vi "Live Capture Functional Stack.vi"() -> ()   [LabVIEW 2013]
uses:
  subvis/Stack Track.ctl
  subvis/Stack_State.ctl
panel:
  in  "Internal Line Interval":dbl
  in  "Slit Width / Lines":sgl=150.0
  in  "Camera Readout Mode":u16(ring)=12 items=["Full Frame"=1, "Slit Scanning"=12]
  in  "Readout Direction":sgl(ring)=1.0 items=["Forward"=1, "Backward"=2]
  in  "Trigger Mode":sgl(ring)=1.0 items=["Normal"=1, "Start "=6]
  in  "Trigger Source":sgl(ring)=2.0 items=["Internal"=1, "External"=2]
  out "Enum":T1
  out "Image":u16[][](graph)
  out "Saving":bool
  in  "AutoIncrement":bool=TRUE
  in  "Path":path=path "C:/Users/spim/Desktop/Craig Cap/temp/a.tiff"
  in  "Frames":i32=100
  out "Frame Index":i32
  out "error out":errorcluster
  in  "stop":bool
  in  "Capture":bool
  out "Total Frames":i32
  out "Elapsed Time":u32
  out "Software FPS":dbl
  out "Camera FPS":dbl
  in  "H Offset":i32 min=0 max=0 step=4
  in  "H Width":i32 min=4 max=2048 step=4
  out "SMD":dbl
  out "SHO":i32
  in  "V Offset":i32 min=0 max=0 step=4
  in  "V Width":i32 min=4 max=2048 step=4
  in  "Binning":u16(ring) items=["1x1"=1, "2x2"=2, "4x4"=4]
  out "SHW":i32
  out "SVO":i32
  out "SVW":i32
  in  "Scan Mode":dbl min=1.0 max=2.0 step=1.0
  in  "Exposure":dbl min=0.0010036691729323308 max=10.000004210526315 step=1e-08
  out "EXP":dbl
  out "Camera Model":string
  out "Camera Version":string
  out "Camera Serial":string
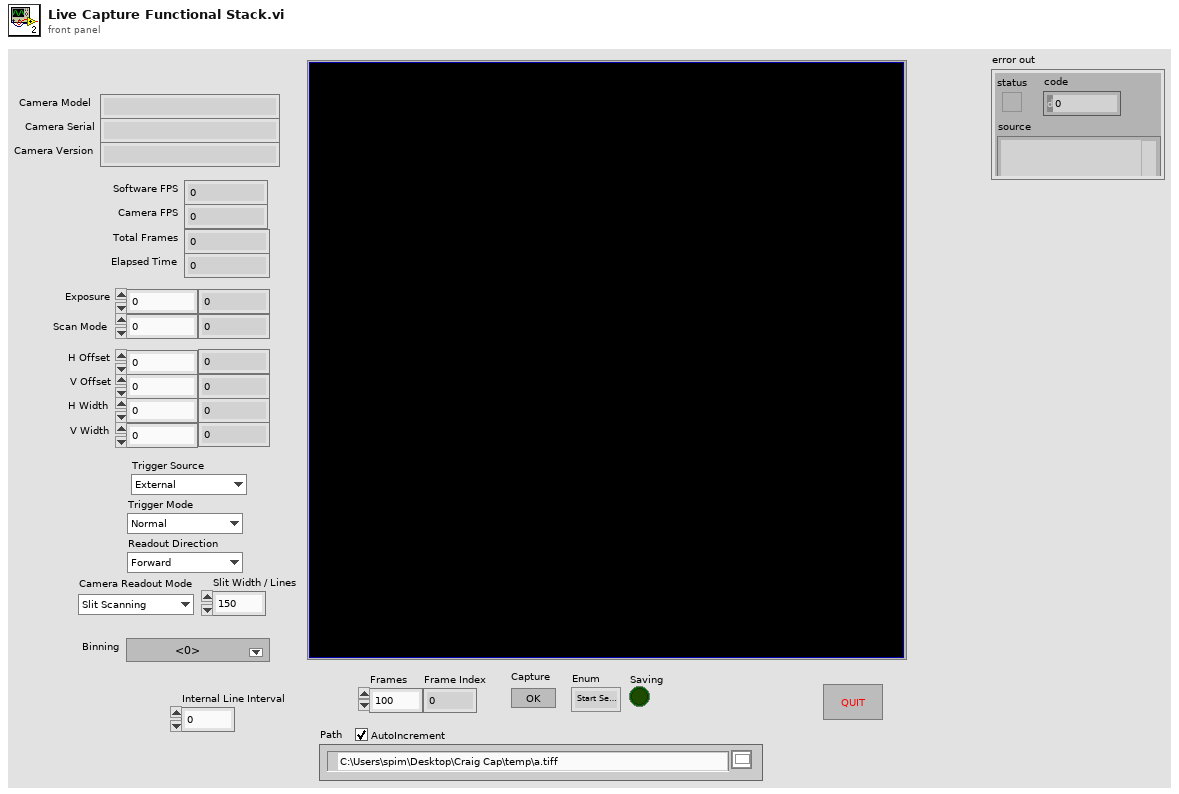
[diagram p1: front panel]
types:
  T1 = typedef "Stack Track.ctl" = enum16{"Start Sequence", "Idle", "STOP", "Collecting", "End"}
  T2 = enum8{"Enabled", "Disabled", "Disabled and Grayed Out"}
  T3 = typedef "Stack_State.ctl" = cluster{"Enum":T1, "Stack Number":i32}
  T4 = cluster{"Model":string, "Camera ID":string, "Firmware":string}
  T5 = cluster{"Value":i32, "Minimum":i32, "Maximum":i32, "Increment":i32}
  T6 = cluster{"height":u32, "width":u32, "datatype":u32}
  T7 = cluster{"H Offset":i32, "V Offset":i32, "H Width":i32, "V Width":i32}
  T8 = typedef "Image Type" = u32
  T9 = typedef "IMAQ Image.ctl" = refnum<image>
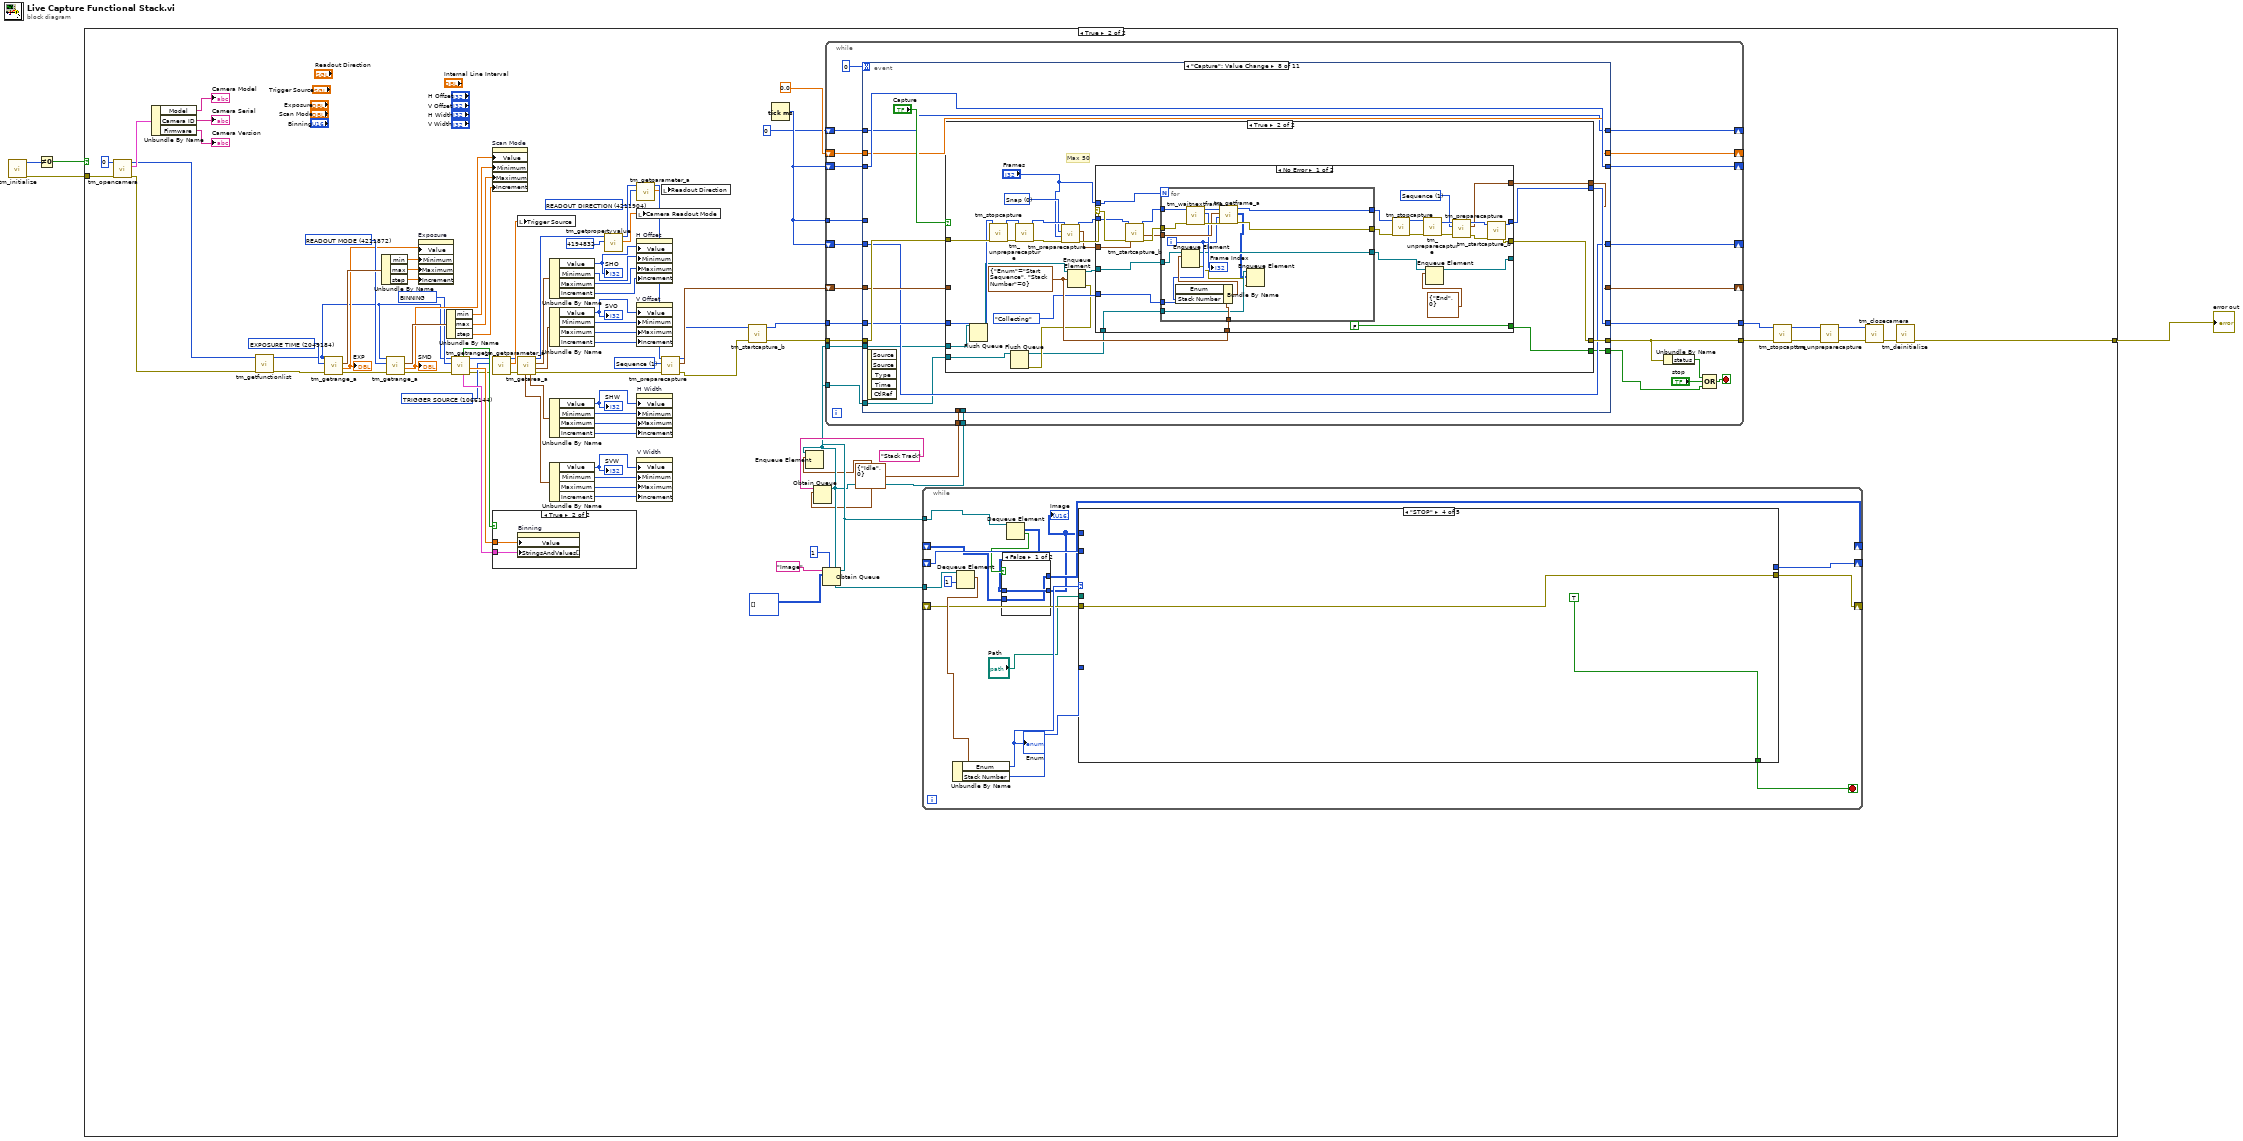
[diagram p0: block diagram]
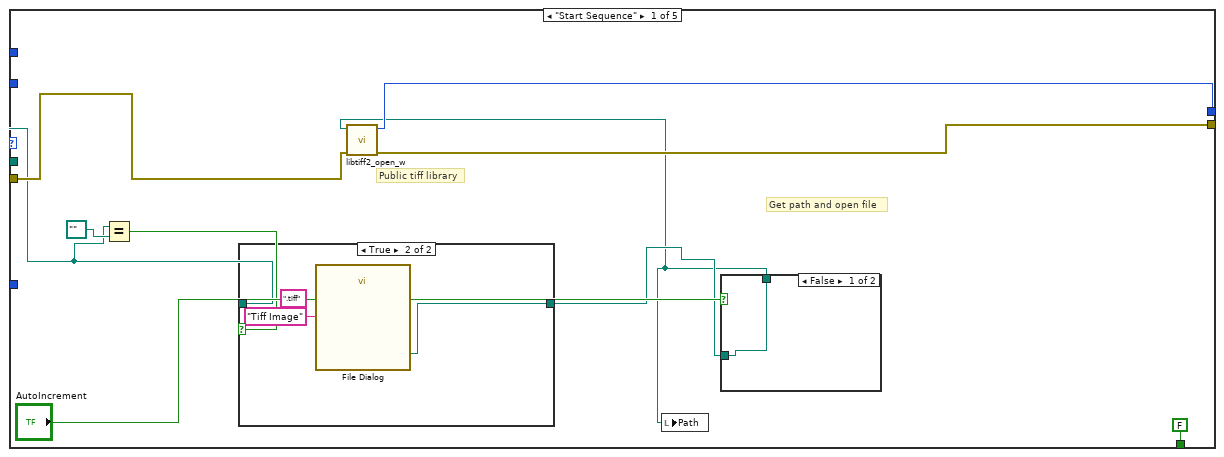
[diagram p4: hidden frame]
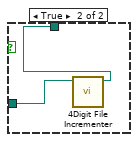
[diagram p6: hidden frame]
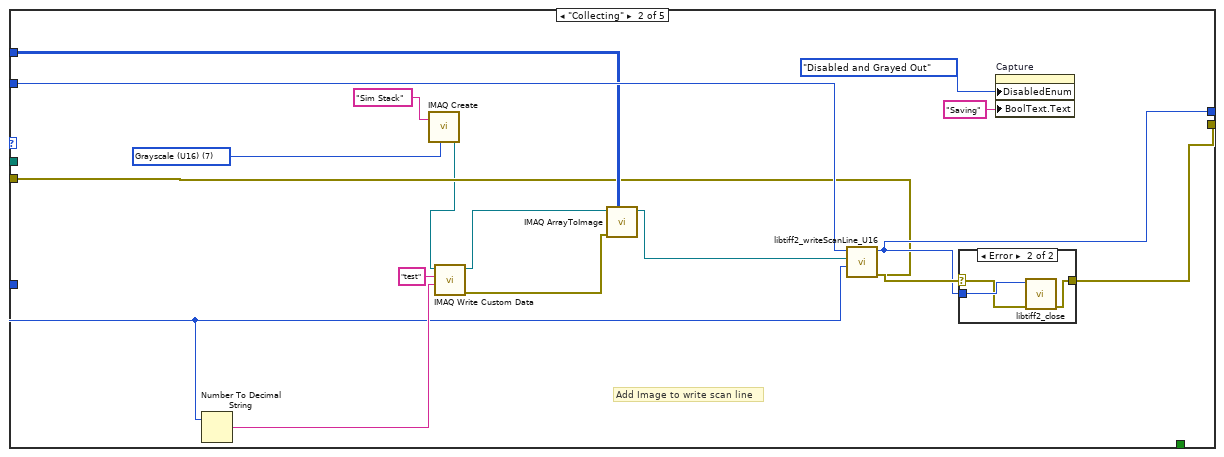
[diagram p7: hidden frame]
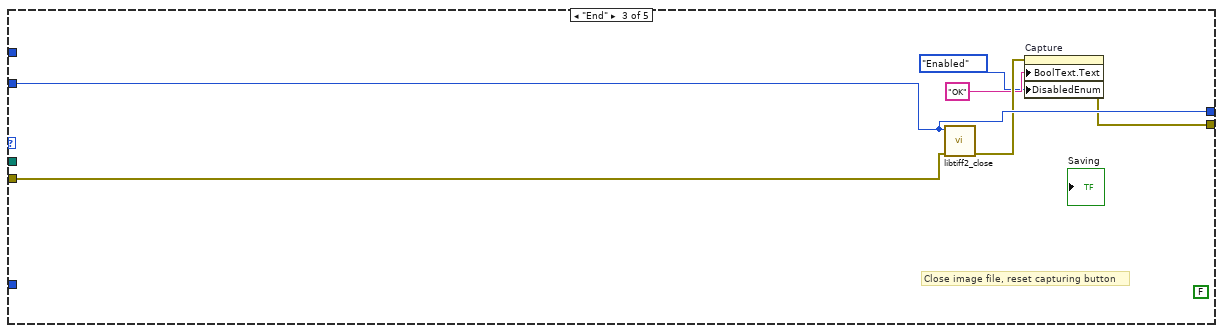
[diagram p9: hidden frame]
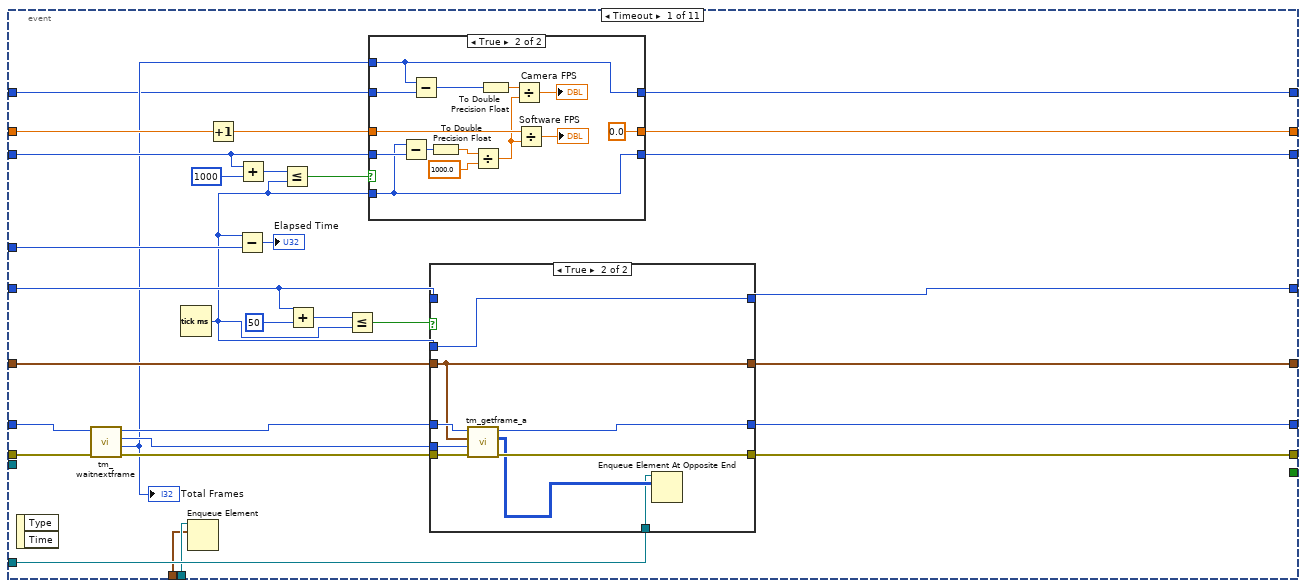
[diagram p12: hidden frame]
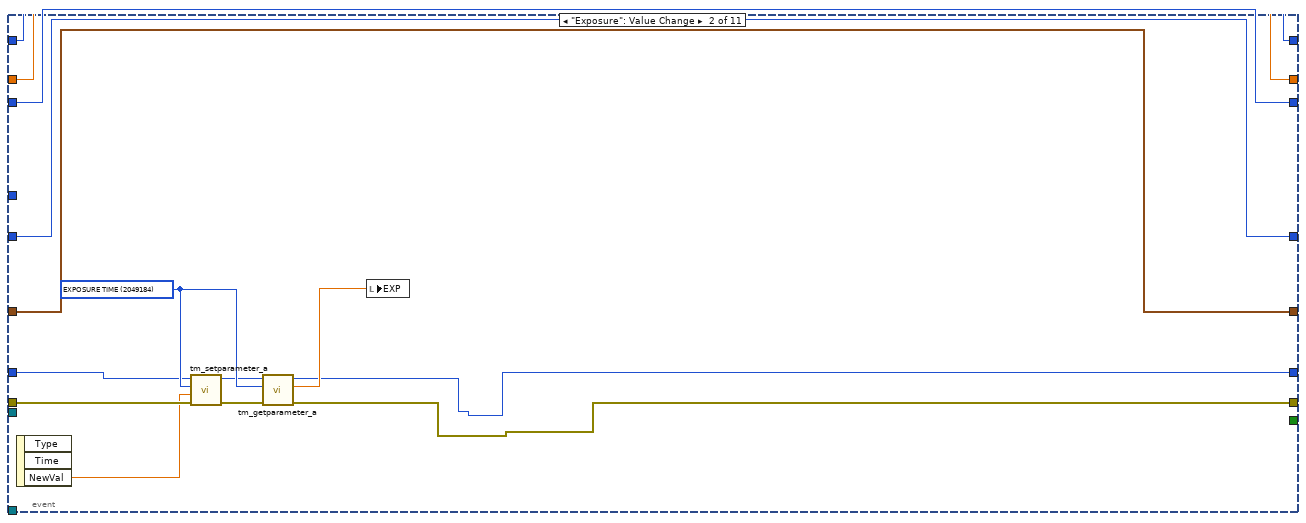
[diagram p15: hidden frame]
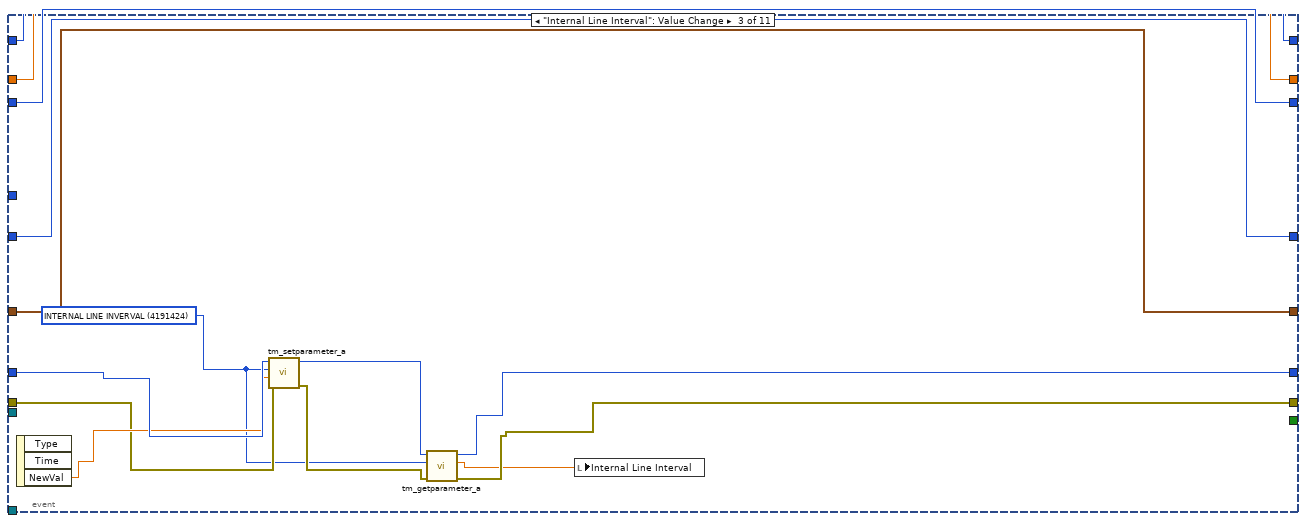
[diagram p16: hidden frame]
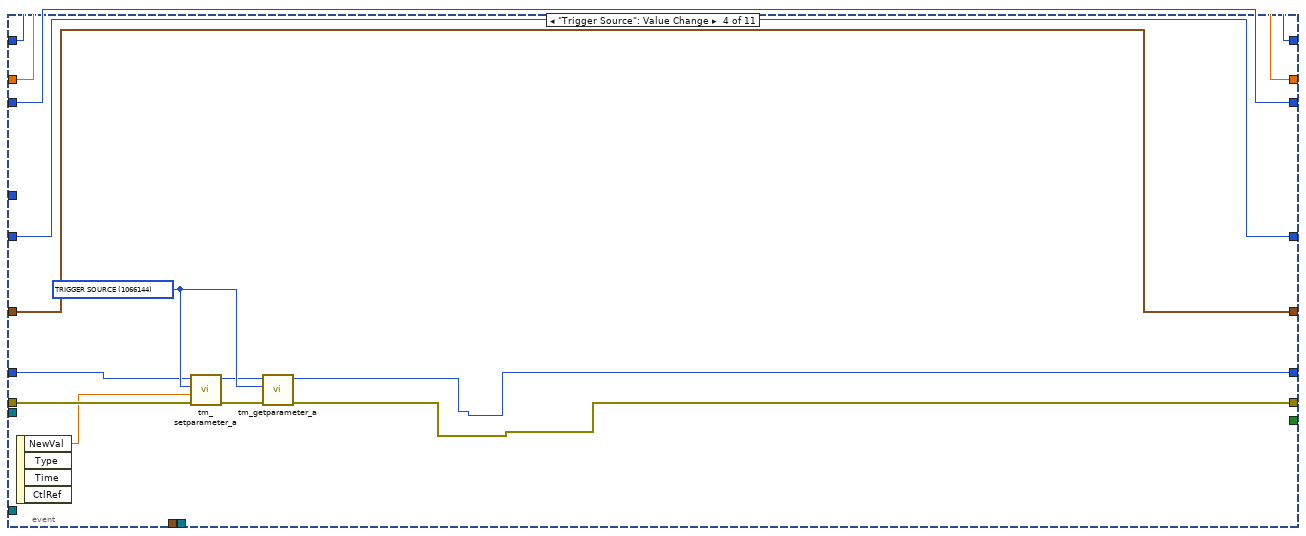
[diagram p17: hidden frame]
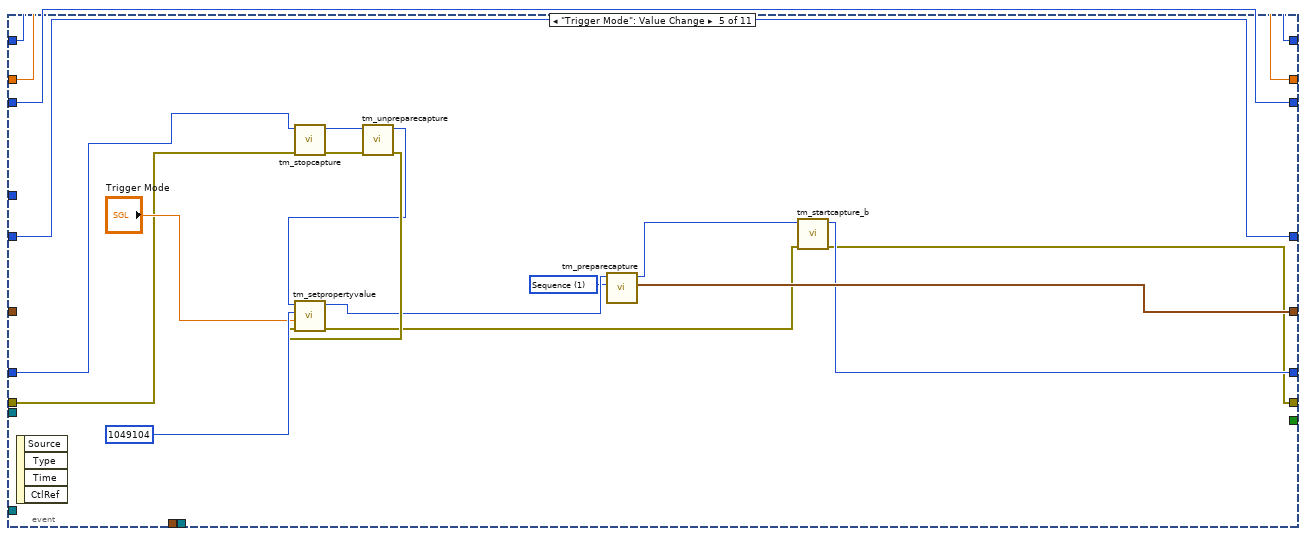
[diagram p18: hidden frame]
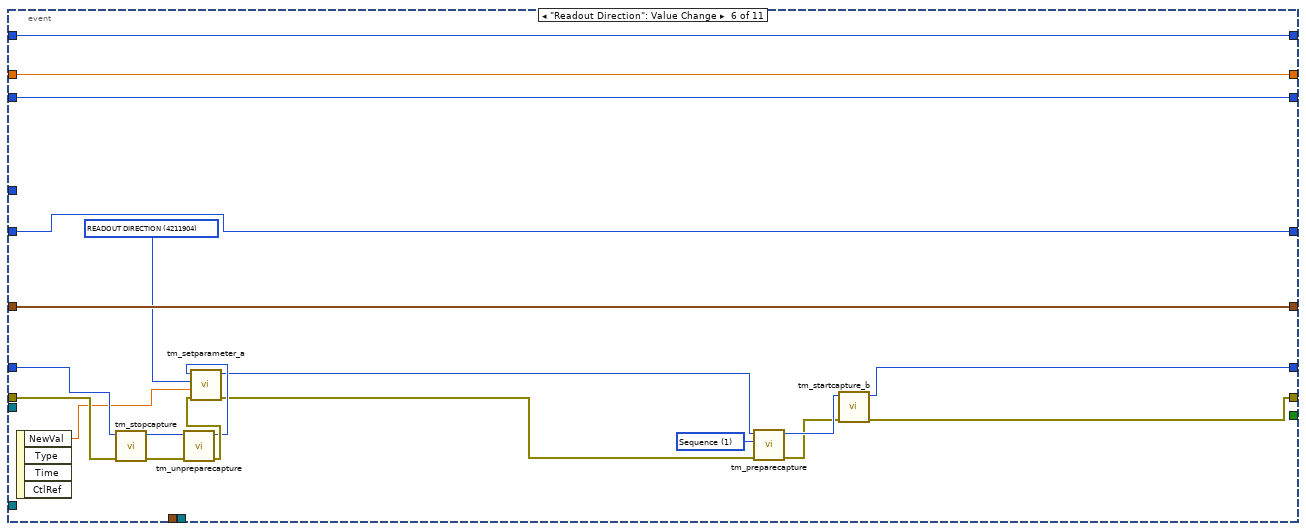
[diagram p19: hidden frame]
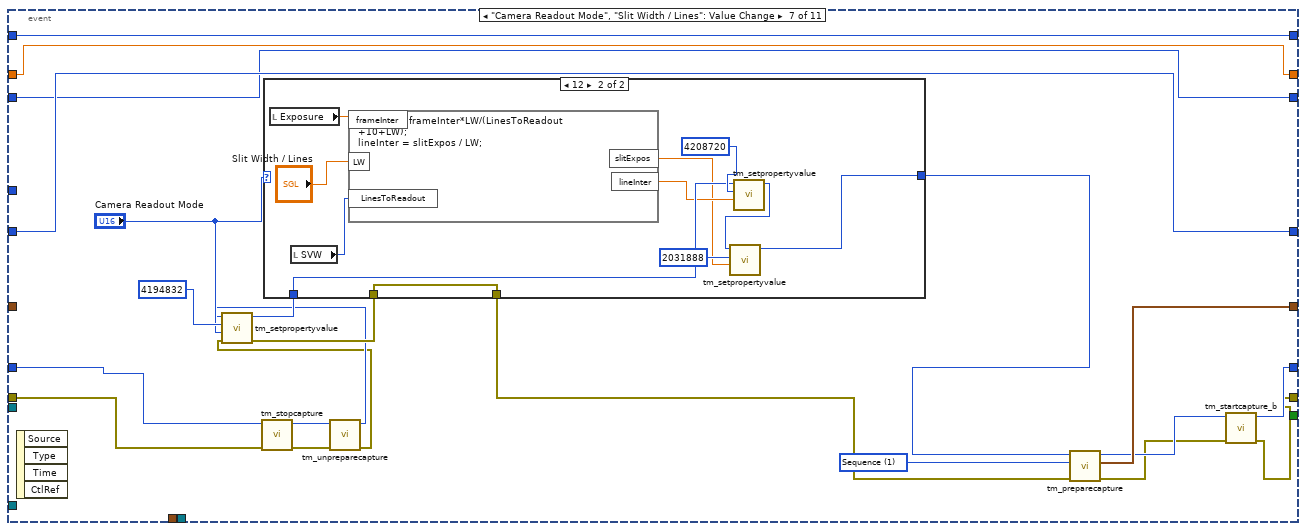
[diagram p20: hidden frame]
diagram:
  n1 = call <userlib>:"tm_initialize.vi"() -> ("error out"=w2:errorcluster, "Number Of Cameras"=w1:u32)  [unwired: 8 in, 2 out]
  n2 = Not Equal To 0?(x=w1) -> (x != 0?=w4:bool)
  n3 = case shown="True" w4 {
    tunnel: [w5 w88] -> w3
    tunnel: w2 -> [w5 w91]
    frame False {
    }
    frame True {
      w10 = u32 4211904 items=["SENSOR MODE"=4212128, "CCD MODE"=4212384, "READOUT MODE"=4211872, "ACTIVE VIEW INDEX"=4343136, "BITS PER CHANNEL"=4342976, "IMAGE PIXEL TYPE"=4343296, "BINNING"=4215968, "EXPOSURE TIME"=2049184, "CONTRAST GAIN"=3163312, "CONTRAST OFFSET"=3163328, "LIGHT MODE"=2114720, "SENSITIVITY"=2114992, "PHOTON IMAGING MODE"=2115200, "HIGH DYNAMIC RANGE MODE"=3163360, "WHITE BALANCE"=3163568, "TEMPERATURE"=2115232, "TEMPERATURE TARGET"=2115264, "SENSOR COOLER FAN"=2115296, "LINEBUNDLE HEIGHT"=4212192, "MECHANICAL SHUTTER"=2115488, "BACK FOCUS POSITION"=8422304, "TRIGGER CONNECTOR"=1066432, "TRIGGER SOURCE"=1066144, "OUTPUT TRIGGER SOURCE"=1852576, "TRIGGER GLOBAL EXPOSURE"=2049680, "FIRST TRIGGER BEHAVIOR"=2049696, "CHANNEL SYNC"=1852352, "READOUT DIRECTION"=4211904, "PRE HSYNC COUNT"=1852704] ("Parameter")
      w20 = u32 1066144 items=["SENSOR MODE"=4212128, "CCD MODE"=4212384, "READOUT MODE"=4211872, "ACTIVE VIEW INDEX"=4343136, "BITS PER CHANNEL"=4342976, "IMAGE PIXEL TYPE"=4343296, "BINNING"=4215968, "EXPOSURE TIME"=2049184, "CONTRAST GAIN"=3163312, "CONTRAST OFFSET"=3163328, "LIGHT MODE"=2114720, "SENSITIVITY"=2114992, "PHOTON IMAGING MODE"=2115200, "HIGH DYNAMIC RANGE MODE"=3163360, "WHITE BALANCE"=3163568, "TEMPERATURE"=2115232, "TEMPERATURE TARGET"=2115264, "SENSOR COOLER FAN"=2115296, "LINEBUNDLE HEIGHT"=4212192, "MECHANICAL SHUTTER"=2115488, "BACK FOCUS POSITION"=8422304, "TRIGGER CONNECTOR"=1066432, "TRIGGER SOURCE"=1066144, "OUTPUT TRIGGER SOURCE"=1852576, "TRIGGER GLOBAL EXPOSURE"=2049680, "FIRST TRIGGER BEHAVIOR"=2049696, "CHANNEL SYNC"=1852352, "READOUT DIRECTION"=4211904, "PRE HSYNC COUNT"=1852704] ("Parameter")
      w27 = T3 {"Enum"=enum."Idle", "Stack Number"=0} ("input cluster")
      w34 = u32 2049184 items=["BINNING"=4215968, "BITS PER CHANNEL"=4342976, "ACTIVE VIEW INDEX"=4343136, "CCD MODE"=4212384, "SENSOR MODE"=4212128, "READOUT MODE"=4211872, "EXPOSURE TIME"=2049184, "CONTRAST GAIN"=3163312, "CONTRAST OFFSET"=3163328, "LIGHT MODE"=2114720, "SENSITIVITY"=2114992, "WHITE BALANCE"=3163568, "PHOTON IMAGING MODE"=2115200, "HIGH DYNAMIC RANGE MODE"=3163360, "TRIGGER SOURCE"=1066144, "TRIGGER ACTIVE"=1066160, "TRIGGER MODE"=1066400, "TRIGGER POLARITY"=1066416, "TRIGGER GLOBAL EXPOSURE"=2049680, "FIRST TRIGGER BEHAVIOR"=2049696, "TRIGGER TIMES"=1066448, "OUTPUT TRIGGER POLARITY"=1852592, "OUTPUT TRIGGER DELAY"=1852624, "OUTPUT TRIGGER PERIOD"=1852640, "TEMPERATURE"=2115232, "TEMPERATURE TARGET"=2115264, "SENSOR COOLER FAN"=2115296, "MECHANICAL SHUTTER"=2115488, "BACK FOCUS POSITION"=8422304, "FRAMEBUNDLE MODE"=4346784, "FRAMEBUNDLE NUMBER"=4346800, "LINEBUNDLE HEIGHT"=4212192, "TRIGGER CONNECTOR"=1066432, "IMAGE PIXEL TYPE"=4343296, "OUTPUT TRIGGER KIND"=1852656, "READOUT DIRECTION"=4211904, "CHANNEL SYNC"=1852352] ("Parameter")
      w35 = u32 4211872 items=["BINNING"=4215968, "BITS PER CHANNEL"=4342976, "ACTIVE VIEW INDEX"=4343136, "CCD MODE"=4212384, "SENSOR MODE"=4212128, "READOUT MODE"=4211872, "EXPOSURE TIME"=2049184, "CONTRAST GAIN"=3163312, "CONTRAST OFFSET"=3163328, "LIGHT MODE"=2114720, "SENSITIVITY"=2114992, "WHITE BALANCE"=3163568, "PHOTON IMAGING MODE"=2115200, "HIGH DYNAMIC RANGE MODE"=3163360, "TRIGGER SOURCE"=1066144, "TRIGGER ACTIVE"=1066160, "TRIGGER MODE"=1066400, "TRIGGER POLARITY"=1066416, "TRIGGER GLOBAL EXPOSURE"=2049680, "FIRST TRIGGER BEHAVIOR"=2049696, "TRIGGER TIMES"=1066448, "OUTPUT TRIGGER POLARITY"=1852592, "OUTPUT TRIGGER DELAY"=1852624, "OUTPUT TRIGGER PERIOD"=1852640, "TEMPERATURE"=2115232, "TEMPERATURE TARGET"=2115264, "SENSOR COOLER FAN"=2115296, "MECHANICAL SHUTTER"=2115488, "BACK FOCUS POSITION"=8422304, "FRAMEBUNDLE MODE"=4346784, "FRAMEBUNDLE NUMBER"=4346800, "LINEBUNDLE HEIGHT"=4212192, "TRIGGER CONNECTOR"=1066432, "IMAGE PIXEL TYPE"=4343296, "OUTPUT TRIGGER KIND"=1852656, "READOUT DIRECTION"=4211904, "CHANNEL SYNC"=1852352] ("Parameter")
      w36 = u32 4215968 items=["BINNING"=4215968, "BITS PER CHANNEL"=4342976, "ACTIVE VIEW INDEX"=4343136, "CCD MODE"=4212384, "SENSOR MODE"=4212128, "READOUT MODE"=4211872, "EXPOSURE TIME"=2049184, "CONTRAST GAIN"=3163312, "CONTRAST OFFSET"=3163328, "LIGHT MODE"=2114720, "SENSITIVITY"=2114992, "WHITE BALANCE"=3163568, "PHOTON IMAGING MODE"=2115200, "HIGH DYNAMIC RANGE MODE"=3163360, "TRIGGER SOURCE"=1066144, "TRIGGER ACTIVE"=1066160, "TRIGGER MODE"=1066400, "TRIGGER POLARITY"=1066416, "TRIGGER GLOBAL EXPOSURE"=2049680, "FIRST TRIGGER BEHAVIOR"=2049696, "TRIGGER TIMES"=1066448, "OUTPUT TRIGGER POLARITY"=1852592, "OUTPUT TRIGGER DELAY"=1852624, "OUTPUT TRIGGER PERIOD"=1852640, "TEMPERATURE"=2115232, "TEMPERATURE TARGET"=2115264, "SENSOR COOLER FAN"=2115296, "MECHANICAL SHUTTER"=2115488, "BACK FOCUS POSITION"=8422304, "FRAMEBUNDLE MODE"=4346784, "FRAMEBUNDLE NUMBER"=4346800, "LINEBUNDLE HEIGHT"=4212192, "TRIGGER CONNECTOR"=1066432, "IMAGE PIXEL TYPE"=4343296, "OUTPUT TRIGGER KIND"=1852656, "READOUT DIRECTION"=4211904, "CHANNEL SYNC"=1852352] ("Parameter")
      w86 = 1 items=["Snap", "Sequence"] ("Capture mode")
      n4 = call <userlib>:"tm_opencamera.vi"("error in (no error)"=w91, "Camera Index"=u32 0) -> ("error out"=w24:errorcluster, "Camera Details"=w48:T4, "Handle out"=w8:u32)  [unwired: 7 in]
      n5 = Unbundle By Name(w48) -> ("Model"=→"Camera Model":string, "Camera ID"=→"Camera Serial":string, "Firmware"=→"Camera Version":string)
      n6 = call <userlib>:"tm_getfunctionlist.vi"("error in (no error)"=w24, "Handle in"=w8) -> ("error out"=w23:errorcluster, "Handle out"=w25:u32)  [unwired: 7 in, 1 out]
      n7 = call <userlib>:"tm_getrange_a.vi"("error in (no error)"=w23, "Parameter"=w34, "Handle in"=w25) -> ("error out"=w43:errorcluster, "default"=w26:dbl, "Range"=w44:cluster{"min":dbl, "max":dbl, "step":dbl})  [unwired: 2 in, 4 out]
      "EXP" <- w26
      n8 = Unbundle By Name(w44) -> ("min"=w81:dbl, "max"=w80:dbl, "step"=w79:dbl)
      n9 = call <userlib>:"tm_getrange_a.vi"("error in (no error)"=w43, "Parameter"=w35, "Handle in"=w25) -> ("error out"=w40:errorcluster, "default"=w41:dbl, "Range"=w42:cluster{"min":dbl, "max":dbl, "step":dbl})  [unwired: 2 in, 4 out]
      "SMD" <- w41
      n10 = property on="Exposure" class="DigNum (strict)"("Value"=w26, "Minimum"=w81, "Maximum"=w80, "Increment"=w79) -> ()  [unwired: 2 in, 2 out]
      n11 = Unbundle By Name(w42) -> ("min"=w78:dbl, "max"=w77:dbl, "step"=w76:dbl)
      n12 = call <userlib>:"tm_getrange_a.vi"("error in (no error)"=w40, "Parameter"=w36, "Handle in"=w25) -> ("error out"=w17:errorcluster, "default"=w38:dbl, "Handle out"=w19:u32, "Value Names"=w37:cluster{"Name":string, "Value":dbl}[], "Writable"=w39:bool)  [unwired: 2 in, 2 out]
      n13 = property on="Scan Mode" class="DigNum (strict)"("Value"=w41, "Minimum"=w78, "Maximum"=w77, "Increment"=w76) -> ()  [unwired: 2 in, 2 out]
      n14 = call <userlib>:"tm_getparameter_a.vi"("error in (no error)"=w17, "Parameter"=w20, "Handle in"=w19) -> ("error out"=w16:errorcluster, "Value out"=w21:dbl, "Handle out"=w18:u32)  [unwired: 6 in]
      n15 = case shown="True" w39 {
        tunnel: w37 -> [_ w161]
        tunnel: w38 -> [_ w160]
        frame False {
        }
        frame True {
          n16 = property on="Binning" class="Ring (strict)"("Value"=w160, "StringsAndValues[]"=w161) -> ()  [unwired: 2 in, 2 out]
        }
      }
      n17 = local write "Trigger Source"(w21) -> ()
      n18 = call <userlib>:"tm_getarea_a.vi"("error in (no error)"=w16, "Handle in"=w18) -> ("error out"=w22:errorcluster, "V Offset"=w75:T5, "H Offset"=w54:T5, "Handle out"=w13:u32, "H Width"=w74:T5, "V Width"=w73:T5)  [unwired: 4 in]
      n19 = Unbundle By Name(w54) -> ("Value"=w53:i32, "Minimum"=w52:i32, "Maximum"=w51:i32, "Increment"=w50:i32)
      "SHO" <- w53
      n20 = Unbundle By Name(w75) -> ("Value"=w63:i32, "Minimum"=w72:i32, "Maximum"=w71:i32, "Increment"=w70:i32)
      "SVO" <- w63
      n21 = Unbundle By Name(w74) -> ("Value"=w62:i32, "Minimum"=w69:i32, "Maximum"=w68:i32, "Increment"=w67:i32)
      "SHW" <- w62
      n22 = Unbundle By Name(w73) -> ("Value"=w61:i32, "Minimum"=w66:i32, "Maximum"=w65:i32, "Increment"=w64:i32)
      "SVW" <- w61
      n23 = call <userlib>:"tm_getpropertyvalue.vi"("Property ID"=u32 4194832, "Handle in"=w13) -> ("Value in"=w14:sgl, "Handle out"=w12:u32)  [unwired: 7 in, 1 out]
      n24 = call <userlib>:"tm_getparameter_a.vi"("Parameter"=w10, "Handle in"=w12) -> ("Value out"=w9:dbl, "Handle out"=w11:u32)  [unwired: 7 in, 1 out]
      n25 = local write "Camera Readout Mode"(w14) -> ()
      n26 = property on="H Offset" class="DigNum (strict)"("Value"=w53, "Minimum"=w52, "Maximum"=w51, "Increment"=w50) -> ()  [unwired: 2 in, 2 out]
      n27 = property on="V Offset" class="DigNum (strict)"("Value"=w63, "Minimum"=w72, "Maximum"=w71, "Increment"=w70) -> ()  [unwired: 2 in, 2 out]
      n28 = property on="H Width" class="DigNum (strict)"("Value"=w62, "Minimum"=w69, "Maximum"=w68, "Increment"=w67) -> ()  [unwired: 2 in, 2 out]
      n29 = property on="V Width" class="DigNum (strict)"("Value"=w61, "Minimum"=w66, "Maximum"=w65, "Increment"=w64) -> ()  [unwired: 2 in, 2 out]
      n30 = local write "Readout Direction"(w9) -> ()
      n31 = call <userlib>:"tm_preparecapture.vi"("error in (no error)"=w22, "Capture mode"=w86, "Handle in"=w11) -> ("error out"=w6:errorcluster, "Buffer Info"=w83:T6, "Handle out"=w7:u32)  [unwired: 5 in, 1 out]
      n32 = call <userlib>:"tm_startcapture_b.vi"("error in (no error)"=w6, "Handle in"=w7) -> ("error out"=w85:errorcluster, "Handle out"=w84:u32)  [unwired: 8 in]
      n33 = Tick Count (ms)() -> (millisecond timer value=w82:u32)
      n34 = Obtain Queue(name (unnamed)="Stack Track", element data type=w27) -> (queue out=w28:refnum<queue>)  [unwired: 3 in, 2 out]
      n35 = Enqueue Element(queue=w28, element=w27) -> ()  [unwired: 2 in, 3 out]
      n36 = Obtain Queue(max queue size (-1, unlimited)=1, name (unnamed)="Image", element data type=u16[][] []) -> (queue out=w29:refnum<queue>)  [unwired: 2 in, 2 out]
      n37 = while {
        tunnel: w85 -> [w174]
        tunnel: [w172] -> w60
        tunnel: [w171] -> w59
        shift-right: [w181] -> _
        shift-left: w82 -> [w179]
        shift-right: [w182] -> _
        shift-left: 0.0 -> [w180]
        shift-right: [w173] -> _
        shift-left: w82 -> [w177]
        tunnel: w84 -> [w175]
        tunnel: w82 -> [w178]
        shift-right: [w170] -> _
        shift-left: w83 -> [w176]
        shift-right: [w167] -> _
        shift-left: 0 -> [w168]
        tunnel: w29 -> [w165]
        tunnel: w28 -> [w166]
        tunnel: w28 -> [w164]
        tunnel: w27 -> [w163]
        stop <- w183 stop-if-true
        n38 = event shown="[7] \"Capture\": Value Change" {
          selector: _ -> [_ _ _ _ _ _ _ _ _ _ _]
          dyn-events: _ -> [_ _ _ _ _ _ _ _ _ _ _]
          timeout: 0 -> [_ _ _ _ _ _ _ _ _ _ _]
          tunnel: [w194 w258 w272 w285 w304 w324 w346 w373 w486 w522 w567] -> w182
          tunnel: [w193 w259 w273 w286 w305 w325 w347 w374 w487 w523 w568] -> w181
          tunnel: w180 -> [w205 w258 w272 w285 w304 w324 w346 w373 w486 w522 w567]
          tunnel: w179 -> [w196 w259 w273 w286 w305 w325 w347 w374 w487 w523 w568]
          tunnel: w178 -> [w201 _ _ _ _ _ _ _ _ _ _]
          tunnel: w177 -> [w206 w260 w274 w287 w306 w326 w348 w369 w488 w530 w575]
          tunnel: w176 -> [w200 w257 w271 w284 _ w323 _ w370 _ _ _]
          tunnel: w175 -> [w208 w252 w266 w280 w298 w317 w339 w377 w483 w499 w537]
          tunnel: w174 -> [w207 w254 w262 w281 w297 w320 w338 w378 w482 w498 w536]
          tunnel: [w204 w260 w274 w287 w306 w326 w348 w369 w488 w530 w575] -> w173
          tunnel: [w203 w248 w269 w277 w289 w310 w329 w375 w477 w525 w570] -> w172
          tunnel: [w202 w247 w268 w276 w288 w309 w327 w376 w478 w526 w571] -> w171
          tunnel: [w199 w257 w271 w284 w292 w323 w334 w371 w476 w524 w569] -> w170
          tunnel: w168 -> [w191 w256 w270 w283 w303 w322 w345 w372 w475 w495 w531]
          tunnel: [w190 w256 w270 w283 w303 w322 w345 w372 w475 w495 w531] -> w167
          tunnel: w165 -> [w188 _ _ _ _ _ _ w367 _ _ _]
          tunnel: w166 -> [_ _ _ _ _ _ _ w368 _ _ _]
          tunnel: w164 -> [w187 _ _ _ _ _ _ _ _ _ _]
          tunnel: w163 -> [w186 _ _ _ _ _ _ _ _ _ _]
          tunnel: [_ _ _ _ _ _ _ w366 _ _ _] -> w162
          event Timeout {
            n39 = event-data() -> ()  [unwired: 1 in, 2 out]
            n40 = call <userlib>:"tm_waitnextframe.vi"("error in (no error)"=w207, "Handle in"=w208) -> ("error out"=w211:errorcluster, "Frame Count"=w192:i32, "Frame Index"=w210:i32, "Handle out"=w212:u32)  [unwired: 6 in]
            "Total Frames" <- w192
            n41 = Tick Count (ms)() -> (millisecond timer value=w198:u32)
            n42 = Enqueue Element(queue=w187, element=w186) -> ()  [unwired: 2 in, 3 out]
            n43 = Increment(x=w205) -> (x+1=w195:dbl)
            n44 = Subtract(x=w198, y=w201) -> (x-y=→"Elapsed Time":u32)
            n45 = Add(x=w196, y=u32 1000) -> (x+y=w216:u32)
            n46 = Less Or Equal?(x=w216, y=w198) -> (x <= y?=w197:bool)
            n47 = Add(x=w206, y=u32 50) -> (x+y=w214:u32)
            n48 = Less Or Equal?(x=w214, y=w198) -> (x <= y?=w189:bool)
            n49 = case shown="True" w197 {
              tunnel: w196 -> [w219 w228]
              tunnel: [w219 w225] -> w193
              tunnel: w195 -> [w218 w231]
              tunnel: w198 -> [_ w225]
              tunnel: [w218 0.0] -> w194
              tunnel: w192 -> [_ w220]
              tunnel: w191 -> [w217 w223]
              tunnel: [w217 w220] -> w190
              frame False {
              }
              frame True {
                n50 = Subtract(x=w225, y=w228) -> (x-y=w227:u32)
                n51 = Subtract(x=w220, y=w223) -> (x-y=w221:i32)
                n52 = To Double Precision Float(number=w227) -> (double precision float=w233:dbl)
                n53 = Divide(x=w233, y=1000.0) -> (x/y=w224:dbl)
                n54 = To Double Precision Float(number=w221) -> (double precision float=w222:dbl)
                n55 = Divide(x=w222, y=w224) -> (x/y=→"Camera FPS":dbl)
                n56 = Divide(x=w231, y=w224) -> (x/y=→"Software FPS":dbl)
              }
            }
            n57 = case shown="True" w189 {
              tunnel: w206 -> [w237 _]
              tunnel: w198 -> [_ w246]
              tunnel: [w237 w246] -> w204
              tunnel: w212 -> [w236 w245]
              tunnel: w200 -> [w234 w240]
              tunnel: w211 -> [w235 w244]
              tunnel: [w236 w243] -> w203
              tunnel: [w235 w242] -> w202
              tunnel: w210 -> [_ w241]
              tunnel: [w234 w240] -> w199
              tunnel: w188 -> [_ w238]
              frame False {
              }
              frame True {
                n58 = call <userlib>:"tm_getframe_a.vi"("error in (no error)"=w244, "Frame Index"=w241, "Buffer Info"=w240, "Handle in"=w245) -> ("error out"=w242:errorcluster, "Data 16"=w239:u16[][], "Handle out"=w243:u32)  [unwired: 3 in, 2 out]
                n59 = Enqueue Element At Opposite End(queue=w238, element=w239) -> ()  [unwired: 2 in, 3 out]
              }
            }
          }
          event "Exposure": Value Change {
            w255 = u32 2049184 items=["SENSOR MODE"=4212128, "CCD MODE"=4212384, "READOUT MODE"=4211872, "ACTIVE VIEW INDEX"=4343136, "BITS PER CHANNEL"=4342976, "IMAGE PIXEL TYPE"=4343296, "BINNING"=4215968, "EXPOSURE TIME"=2049184, "CONTRAST GAIN"=3163312, "CONTRAST OFFSET"=3163328, "LIGHT MODE"=2114720, "SENSITIVITY"=2114992, "PHOTON IMAGING MODE"=2115200, "HIGH DYNAMIC RANGE MODE"=3163360, "WHITE BALANCE"=3163568, "TEMPERATURE"=2115232, "TEMPERATURE TARGET"=2115264, "SENSOR COOLER FAN"=2115296, "LINEBUNDLE HEIGHT"=4212192, "MECHANICAL SHUTTER"=2115488, "BACK FOCUS POSITION"=8422304, "TRIGGER CONNECTOR"=1066432, "TRIGGER SOURCE"=1066144, "OUTPUT TRIGGER SOURCE"=1852576, "TRIGGER GLOBAL EXPOSURE"=2049680, "FIRST TRIGGER BEHAVIOR"=2049696, "CHANNEL SYNC"=1852352, "READOUT DIRECTION"=4211904, "PRE HSYNC COUNT"=1852704] ("Parameter")
            n60 = event-data() -> ("NewVal"=w253:dbl)  [unwired: 1 in, 2 out]
            n61 = call <userlib>:"tm_setparameter_a.vi"("error in (no error)"=w254, "Value in"=w253, "Parameter"=w255, "Handle in"=w252) -> ("error out"=w251:errorcluster, "Handle out"=w250:u32)  [unwired: 6 in]
            n62 = call <userlib>:"tm_getparameter_a.vi"("error in (no error)"=w251, "Parameter"=w255, "Handle in"=w250) -> ("error out"=w247:errorcluster, "Value out"=w249:dbl, "Handle out"=w248:u32)  [unwired: 6 in]
            n63 = local write "EXP"(w249) -> ()
          }
          event "Internal Line Interval": Value Change {
            w261 = u32 4191424 items=["SENSOR MODE"=4212128, "CCD MODE"=4212384, "READOUT MODE"=4211872, "ACTIVE VIEW INDEX"=4343136, "BITS PER CHANNEL"=4342976, "IMAGE PIXEL TYPE"=4343296, "BINNING"=4215968, "EXPOSURE TIME"=2049184, "CONTRAST GAIN"=3163312, "CONTRAST OFFSET"=3163328, "LIGHT MODE"=2114720, "SENSITIVITY"=2114992, "PHOTON IMAGING MODE"=2115200, "HIGH DYNAMIC RANGE MODE"=3163360, "WHITE BALANCE"=3163568, "TEMPERATURE"=2115232, "TEMPERATURE TARGET"=2115264, "SENSOR COOLER FAN"=2115296, "LINEBUNDLE HEIGHT"=4212192, "MECHANICAL SHUTTER"=2115488, "BACK FOCUS POSITION"=8422304, "TRIGGER CONNECTOR"=1066432, "TRIGGER SOURCE"=1066144, "OUTPUT TRIGGER SOURCE"=1852576, "TRIGGER GLOBAL EXPOSURE"=2049680, "FIRST TRIGGER BEHAVIOR"=2049696, "CHANNEL SYNC"=1852352, "READOUT DIRECTION"=4211904, "PRE HSYNC COUNT"=1852704, "INTERNAL LINE SPEED"=4191408, "INTERNAL LINE INVERVAL"=4191424] ("Parameter")
            n64 = event-data() -> ("NewVal"=w265:dbl)  [unwired: 1 in, 2 out]
            n65 = call <userlib>:"tm_setparameter_a.vi"("error in (no error)"=w262, "Value in"=w265, "Parameter"=w261, "Handle in"=w266) -> ("error out"=w263:errorcluster, "Handle out"=w264:u32)  [unwired: 6 in]
            n66 = call <userlib>:"tm_getparameter_a.vi"("error in (no error)"=w263, "Parameter"=w261, "Handle in"=w264) -> ("error out"=w268:errorcluster, "Value out"=w267:dbl, "Handle out"=w269:u32)  [unwired: 6 in]
            n67 = local write "Internal Line Interval"(w267) -> ()
          }
          event "Trigger Source": Value Change {
            w282 = u32 1066144 items=["SENSOR MODE"=4212128, "CCD MODE"=4212384, "READOUT MODE"=4211872, "ACTIVE VIEW INDEX"=4343136, "BITS PER CHANNEL"=4342976, "IMAGE PIXEL TYPE"=4343296, "BINNING"=4215968, "EXPOSURE TIME"=2049184, "CONTRAST GAIN"=3163312, "CONTRAST OFFSET"=3163328, "LIGHT MODE"=2114720, "SENSITIVITY"=2114992, "PHOTON IMAGING MODE"=2115200, "HIGH DYNAMIC RANGE MODE"=3163360, "WHITE BALANCE"=3163568, "TEMPERATURE"=2115232, "TEMPERATURE TARGET"=2115264, "SENSOR COOLER FAN"=2115296, "LINEBUNDLE HEIGHT"=4212192, "MECHANICAL SHUTTER"=2115488, "BACK FOCUS POSITION"=8422304, "TRIGGER CONNECTOR"=1066432, "TRIGGER SOURCE"=1066144, "OUTPUT TRIGGER SOURCE"=1852576, "TRIGGER GLOBAL EXPOSURE"=2049680, "FIRST TRIGGER BEHAVIOR"=2049696, "CHANNEL SYNC"=1852352, "READOUT DIRECTION"=4211904, "PRE HSYNC COUNT"=1852704] ("Parameter")
            n68 = event-data() -> ("NewVal"=w275:sgl)  [unwired: 1 in, 3 out]
            n69 = call <userlib>:"tm_setparameter_a.vi"("error in (no error)"=w281, "Value in"=w275, "Parameter"=w282, "Handle in"=w280) -> ("error out"=w279:errorcluster, "Handle out"=w278:u32)  [unwired: 6 in]
            n70 = call <userlib>:"tm_getparameter_a.vi"("error in (no error)"=w279, "Parameter"=w282, "Handle in"=w278) -> ("error out"=w276:errorcluster, "Handle out"=w277:u32)  [unwired: 6 in, 1 out]
          }
          event "Trigger Mode": Value Change {
            w293 = 1 items=["Snap", "Sequence"] ("Capture mode")
            n71 = event-data() -> ()  [unwired: 1 in, 4 out]
            n72 = call <userlib>:"tm_stopcapture.vi"("error in (no error)"=w297, "Handle in"=w298) -> ("error out"=w300:errorcluster, "Handle out"=w299:u32)  [unwired: 8 in]
            n73 = call <userlib>:"tm_unpreparecapture.vi"("error in (no error)"=w300, "Handle in"=w299) -> ("error out"=w296:errorcluster, "Handle out"=w295:u32)  [unwired: 8 in]
            n74 = call <userlib>:"tm_setpropertyvalue.vi"("error in (no error)"=w296, "Value in"="Trigger Mode", "Property ID"=u32 1049104, "Handle in"=w295) -> ("error out"=w291:errorcluster, "Handle out"=w294:u32)  [unwired: 6 in]
            n75 = call <userlib>:"tm_preparecapture.vi"("Capture mode"=w293, "Handle in"=w294) -> ("Buffer Info"=w292:T6, "Handle out"=w290:u32)  [unwired: 6 in, 2 out]
            n76 = call <userlib>:"tm_startcapture_b.vi"("error in (no error)"=w291, "Handle in"=w290) -> ("error out"=w288:errorcluster, "Handle out"=w289:u32)  [unwired: 8 in]
          }
          event "Readout Direction": Value Change {
            w315 = 1 items=["Snap", "Sequence"] ("Capture mode")
            w308 = u32 4211904 items=["SENSOR MODE"=4212128, "CCD MODE"=4212384, "READOUT MODE"=4211872, "ACTIVE VIEW INDEX"=4343136, "BITS PER CHANNEL"=4342976, "IMAGE PIXEL TYPE"=4343296, "BINNING"=4215968, "EXPOSURE TIME"=2049184, "CONTRAST GAIN"=3163312, "CONTRAST OFFSET"=3163328, "LIGHT MODE"=2114720, "SENSITIVITY"=2114992, "PHOTON IMAGING MODE"=2115200, "HIGH DYNAMIC RANGE MODE"=3163360, "WHITE BALANCE"=3163568, "TEMPERATURE"=2115232, "TEMPERATURE TARGET"=2115264, "SENSOR COOLER FAN"=2115296, "LINEBUNDLE HEIGHT"=4212192, "MECHANICAL SHUTTER"=2115488, "BACK FOCUS POSITION"=8422304, "TRIGGER CONNECTOR"=1066432, "TRIGGER SOURCE"=1066144, "OUTPUT TRIGGER SOURCE"=1852576, "TRIGGER GLOBAL EXPOSURE"=2049680, "FIRST TRIGGER BEHAVIOR"=2049696, "CHANNEL SYNC"=1852352, "READOUT DIRECTION"=4211904, "PRE HSYNC COUNT"=1852704] ("Parameter")
            n77 = event-data() -> ("NewVal"=w307:sgl)  [unwired: 1 in, 3 out]
            n78 = call <userlib>:"tm_stopcapture.vi"("error in (no error)"=w320, "Handle in"=w317) -> ("error out"=w321:errorcluster, "Handle out"=w316:u32)  [unwired: 8 in]
            n79 = call <userlib>:"tm_unpreparecapture.vi"("error in (no error)"=w321, "Handle in"=w316) -> ("error out"=w319:errorcluster, "Handle out"=w318:u32)  [unwired: 8 in]
            n80 = call <userlib>:"tm_setparameter_a.vi"("error in (no error)"=w319, "Value in"=w307, "Parameter"=w308, "Handle in"=w318) -> ("error out"=w312:errorcluster, "Handle out"=w311:u32)  [unwired: 6 in]
            n81 = call <userlib>:"tm_preparecapture.vi"("error in (no error)"=w312, "Capture mode"=w315, "Handle in"=w311) -> ("error out"=w313:errorcluster, "Handle out"=w314:u32)  [unwired: 5 in, 2 out]
            n82 = call <userlib>:"tm_startcapture_b.vi"("error in (no error)"=w313, "Handle in"=w314) -> ("error out"=w309:errorcluster, "Handle out"=w310:u32)  [unwired: 8 in]
          }
          event "Camera Readout Mode", "Slit Width / Lines": Value Change {
            w332 = 1 items=["Snap", "Sequence"] ("Capture mode")
            n83 = event-data() -> ()  [unwired: 1 in, 4 out]
            n84 = call <userlib>:"tm_stopcapture.vi"("error in (no error)"=w338, "Handle in"=w339) -> ("error out"=w340:errorcluster, "Handle out"=w336:u32)  [unwired: 8 in]
            n85 = call <userlib>:"tm_unpreparecapture.vi"("error in (no error)"=w340, "Handle in"=w336) -> ("error out"=w331:errorcluster, "Handle out"=w337:u32)  [unwired: 8 in]
            n86 = call <userlib>:"tm_setpropertyvalue.vi"("error in (no error)"=w331, "Value in"="Camera Readout Mode", "Property ID"=u32 4194832, "Handle in"=w337) -> ("error out"=w341:errorcluster, "Handle out"=w342:u32)  [unwired: 6 in]
            n87 = case shown="12" "Camera Readout Mode" {
              tunnel: w342 -> [w353 w360]
              tunnel: [w352 w355] -> w335
              tunnel: w341 -> [w350 w365]
              tunnel: [w349 w365] -> w333
              frame 1, Default {
                n88 = local read "Exposure"() -> (w351:dbl)
                n89 = call <userlib>:"tm_setpropertyvalue.vi"("error in (no error)"=w350, "Value in"=w351, "Property ID"=u32 2031888, "Handle in"=w353) -> ("error out"=w349:errorcluster, "Handle out"=w352:u32)  [unwired: 6 in]
              }
              frame 12 {
                n90 = local read "Exposure"() -> (w364:dbl)
                n91 = local read "SVW"() -> (w362:i32)
                n92 = formula code="slitExpos=frameInter*LW/(LinesToReadout\n+10+LW);\nlineInter = slitExpos / LW;"("frameInter"=w364, "LW"="Slit Width / Lines", "LinesToReadout"=w362) -> ("slitExpos"=w356:dbl, "lineInter"=w359:dbl)
                n93 = call <userlib>:"tm_setpropertyvalue.vi"("Value in"=w359, "Property ID"=u32 4208720, "Handle in"=w360) -> ("Handle out"=w358:u32)  [unwired: 7 in, 1 out]
                n94 = call <userlib>:"tm_setpropertyvalue.vi"("Value in"=w356, "Property ID"=u32 2031888, "Handle in"=w358) -> ("Handle out"=w355:u32)  [unwired: 7 in, 1 out]
              }
            }
            n95 = call <userlib>:"tm_preparecapture.vi"("error in (no error)"=w333, "Capture mode"=w332, "Handle in"=w335) -> ("error out"=w328:errorcluster, "Buffer Info"=w334:T6, "Handle out"=w330:u32)  [unwired: 5 in, 1 out]
            n96 = call <userlib>:"tm_startcapture_b.vi"("error in (no error)"=w328, "Handle in"=w330) -> ("error out"=w327:errorcluster, "Handle out"=w329:u32)  [unwired: 8 in]
          }
          event "Capture": Value Change {
            n97 = event-data() -> ()  [unwired: 1 in, 5 out]
            n98 = case shown="True" "Capture" {
              tunnel: w378 -> [w382 w405]
              tunnel: w377 -> [w381 w402]
              tunnel: [w382 w383] -> w376
              tunnel: [w381 w385] -> w375
              tunnel: [w380 w384] -> w371
              tunnel: w370 -> [w380 _]
              tunnel: w368 -> [_ w391]
              tunnel: w367 -> [_ w388]
              tunnel: [_ w386] -> w366
              frame False {
              }
              frame True {
                w393 = T3 {"Enum"=enum."Start Sequence", "Stack Number"=0} ("input cluster")
                w399 = 0 items=["Snap", "Sequence"] ("Capture mode")
                # "Max 50"
                n99 = Flush Queue(queue=w391) -> (queue out=w390:refnum<queue>)  [unwired: 1 in, 2 out]
                n100 = call <userlib>:"tm_stopcapture.vi"("error in (no error)"=w405, "Handle in"=w402) -> ("error out"=w404:errorcluster, "Handle out"=w403:u32)  [unwired: 8 in]
                n101 = call <userlib>:"tm_unpreparecapture.vi"("error in (no error)"=w404, "Handle in"=w403) -> ("error out"=w400:errorcluster, "Handle out"=w401:u32)  [unwired: 8 in]
                n102 = call <userlib>:"tm_preparecapture.vi"("error in (no error)"=w400, "Frames"="Frames", "Capture mode"=w399, "Handle in"=w401) -> ("error out"=w398:errorcluster, "Buffer Info"=w396:T6, "Handle out"=w397:u32)  [unwired: 4 in, 1 out]
                n103 = Enqueue Element(queue=w390, element=w393) -> (queue out=w394:refnum<queue>, error out=w389:errorcluster)  [unwired: 2 in, 1 out]
                n104 = Flush Queue(queue=w388, error in (no error)=w389) -> (queue out=w387:refnum<queue>)  [unwired: 2 out]
                n105 = case shown="No Error" w398 {
                  selector: w398 -> [w431 w454]
                  tunnel: w397 -> [w430 w455]
                  tunnel: "Frames" -> [w426 _]
                  tunnel: [w409 w451] -> w385
                  tunnel: w396 -> [w427 _]
                  tunnel: [w408 w453] -> w383
                  tunnel: w394 -> [w425 w449]
                  tunnel: w393 -> [w424 _]
                  tunnel: Stack_Track."Collecting" ("Enum") -> [w423 _]
                  tunnel: [w407 w449] -> _
                  tunnel: w387 -> [w422 _]
                  tunnel: [FALSE ("value") w463] -> w386
                  tunnel: [w406 w452] -> w384
                  frame No Error {
                    w414 = 1 items=["Snap", "Sequence"] ("Capture mode")
                    n106 = call <userlib>:"tm_startcapture_b.vi"("error in (no error)"=w431, "Handle in"=w430) -> ("error out"=w428:errorcluster, "Handle out"=w429:u32)  [unwired: 8 in]
                    n107 = for {
                      N: w426 -> [_]
                      tunnel: w429 -> [w448]
                      tunnel: w428 -> [w447]
                      tunnel: w427 -> [w444]
                      tunnel: [w443] -> w420
                      tunnel: [w442] -> w419
                      tunnel: w425 -> [w440]
                      tunnel: w423 -> [w438]
                      tunnel: w424 -> [w436]
                      tunnel: [w435] -> w413
                      tunnel: w422 -> [w434]
                      i -> [w437]
                      n108 = Bundle By Name(cluster=w436, "Enum"=w438, "Stack Number"=w437) -> (w439:T3)
                      n109 = Enqueue Element(queue=w440, element=w439) -> (queue out=w435:refnum<queue>, error out=w432:errorcluster)  [unwired: 2 in, 1 out]
                      n110 = call <userlib>:"tm_waitnextframe.vi"("error in (no error)"=w447, "Handle in"=w448) -> ("error out"=w445:errorcluster, "Frame Index"=→"Frame Index":i32, "Handle out"=w446:u32)  [unwired: 6 in, 1 out]
                      n111 = call <userlib>:"tm_getframe_a.vi"("error in (no error)"=w445, "Frame Index"=w437, "Buffer Info"=w444, "Handle in"=w446) -> ("error out"=w442:errorcluster, "Data 16"=w433:u16[][], "Handle out"=w443:u32)  [unwired: 3 in, 2 out]
                      n112 = Enqueue Element(queue=w434, element=w433, error in (no error)=w432) -> ()  [unwired: 1 in, 3 out]
                    }
                    n113 = call <userlib>:"tm_stopcapture.vi"("error in (no error)"=w419, "Handle in"=w420) -> ("error out"=w417:errorcluster, "Handle out"=w418:u32)  [unwired: 8 in]
                    n114 = call <userlib>:"tm_unpreparecapture.vi"("error in (no error)"=w417, "Handle in"=w418) -> ("error out"=w416:errorcluster, "Handle out"=w415:u32)  [unwired: 8 in]
                    n115 = Enqueue Element(queue=w413, element=T3 {"Enum"=enum."End", "Stack Number"=0} ("input cluster")) -> (queue out=w407:refnum<queue>)  [unwired: 2 in, 2 out]
                    n116 = call <userlib>:"tm_preparecapture.vi"("error in (no error)"=w416, "Capture mode"=w414, "Handle in"=w415) -> ("error out"=w411:errorcluster, "Buffer Info"=w406:T6, "Handle out"=w410:u32)  [unwired: 5 in, 1 out]
                    n117 = call <userlib>:"tm_startcapture_b.vi"("error in (no error)"=w411, "Handle in"=w410) -> ("error out"=w408:errorcluster, "Handle out"=w409:u32)  [unwired: 8 in]
                  }
                  frame Error {
                    w458 = 1 items=["Snap", "Sequence"] ("Capture mode")
                    # "Prepare camera failure, likely too many frames in stack"
                    n118 = One Button Dialog(message="Too many frames in stack", button name ("OK")="OK") -> (true=w463:bool)
                    n119 = call <userlib>:"tm_stopcapture.vi"("error in (no error)"=w454, "Handle in"=w455) -> ("error out"=w461:errorcluster, "Handle out"=w462:u32)  [unwired: 8 in]
                    n120 = call <userlib>:"tm_unpreparecapture.vi"("error in (no error)"=w461, "Handle in"=w462) -> ("error out"=w460:errorcluster, "Handle out"=w459:u32)  [unwired: 8 in]
                    n121 = Enqueue Element(queue=w449, element=T3 {"Enum"=enum."STOP", "Stack Number"=0} ("input cluster")) -> ()  [unwired: 2 in, 3 out]
                    n122 = call <userlib>:"tm_preparecapture.vi"("error in (no error)"=w460, "Capture mode"=w458, "Handle in"=w459) -> ("error out"=w457:errorcluster, "Buffer Info"=w452:T6, "Handle out"=w456:u32)  [unwired: 5 in, 1 out]
                    n123 = call <userlib>:"tm_startcapture_b.vi"("error in (no error)"=w457, "Handle in"=w456) -> ("error out"=w453:errorcluster, "Handle out"=w451:u32)  [unwired: 8 in]
                  }
                }
              }
            }
          }
          event "Scan Mode": Value Change {
            w466 = u32 4211872 items=["SENSOR MODE"=4212128, "CCD MODE"=4212384, "READOUT MODE"=4211872, "ACTIVE VIEW INDEX"=4343136, "BITS PER CHANNEL"=4342976, "IMAGE PIXEL TYPE"=4343296, "BINNING"=4215968, "EXPOSURE TIME"=2049184, "CONTRAST GAIN"=3163312, "CONTRAST OFFSET"=3163328, "LIGHT MODE"=2114720, "SENSITIVITY"=2114992, "PHOTON IMAGING MODE"=2115200, "HIGH DYNAMIC RANGE MODE"=3163360, "WHITE BALANCE"=3163568, "TEMPERATURE"=2115232, "TEMPERATURE TARGET"=2115264, "SENSOR COOLER FAN"=2115296, "LINEBUNDLE HEIGHT"=4212192, "MECHANICAL SHUTTER"=2115488, "BACK FOCUS POSITION"=8422304, "TRIGGER CONNECTOR"=1066432, "TRIGGER SOURCE"=1066144, "OUTPUT TRIGGER SOURCE"=1852576, "TRIGGER GLOBAL EXPOSURE"=2049680, "FIRST TRIGGER BEHAVIOR"=2049696, "CHANNEL SYNC"=1852352, "READOUT DIRECTION"=4211904, "PRE HSYNC COUNT"=1852704] ("Parameter")
            w481 = 1 items=["Snap", "Sequence"] ("Capture mode")
            n124 = event-data() -> ("NewVal"=w471:dbl)  [unwired: 1 in, 2 out]
            n125 = call <userlib>:"tm_stopcapture.vi"("error in (no error)"=w482, "Handle in"=w483) -> ("error out"=w484:errorcluster, "Handle out"=w485:u32)  [unwired: 8 in]
            n126 = call <userlib>:"tm_unpreparecapture.vi"("error in (no error)"=w484, "Handle in"=w485) -> ("error out"=w469:errorcluster, "Handle out"=w470:u32)  [unwired: 8 in]
            n127 = call <userlib>:"tm_setparameter_a.vi"("error in (no error)"=w469, "Value in"=w471, "Parameter"=w466, "Handle in"=w470) -> ("error out"=w468:errorcluster, "Handle out"=w467:u32)  [unwired: 6 in]
            n128 = call <userlib>:"tm_getparameter_a.vi"("error in (no error)"=w468, "Parameter"=w466, "Handle in"=w467) -> ("error out"=w474:errorcluster, "Value out"=w473:dbl, "Handle out"=w472:u32)  [unwired: 6 in]
            n129 = local write "SMD"(w473) -> ()
            n130 = call <userlib>:"tm_preparecapture.vi"("error in (no error)"=w474, "Capture mode"=w481, "Handle in"=w472) -> ("error out"=w479:errorcluster, "Buffer Info"=w476:T6, "Handle out"=w480:u32)  [unwired: 5 in, 1 out]
            n131 = call <userlib>:"tm_startcapture_b.vi"("error in (no error)"=w479, "Handle in"=w480) -> ("error out"=w478:errorcluster, "Handle out"=w477:u32)  [unwired: 8 in]
          }
          event "Binning": Value Change {
            w490 = u32 4215968 items=["BINNING"=4215968, "BITS PER CHANNEL"=2, "ACTIVE VIEW INDEX"=3, "CCD MODE"=4, "SENSOR MODE"=5, "READOUT MODE"=6, "EXPOSURE TIME"=7, "CONTRAST GAIN"=8, "CONTRAST OFFSET"=9, "LIGHT MODE"=10, "SENSITIVITY"=11, "WHITE BALANCE"=12, "PHOTON IMAGING MODE"=13, "HIGH DYNAMIC RANGE MODE"=14, "TRIGGER SOURCE"=15, "TRIGGER ACTIVE"=16, "TRIGGER MODE"=17, "TRIGGER POLARITY"=18, "TRIGGER GLOBAL EXPOSURE"=19, "FIRST TRIGGER BEHAVIOR"=20, "TRIGGER TIMES"=21, "OUTPUT TRIGGER POLARITY"=22, "OUTPUT TRIGGER DELAY"=23, "OUTPUT TRIGGER PERIOD"=24, "TEMPERATURE"=25, "TEMPERATURE TARGET"=26, "SENSOR COOLER FAN"=27, "MECHANICAL SHUTTER"=28, "BACK FOCUS POSITION"=29, "FRAMEBUNDLE MODE"=30, "FRAMEBUNDLE NUMBER"=31, "LINEBUNDLE HEIGHT"=32, "TRIGGER CONNECTOR"=33, "IMAGE PIXEL TYPE"=34, "OUTPUT TRIGGER KIND"=35, "READOUT DIRECTION"=36, "CHANNEL SYNC"=37] ("Parameter")
            w529 = 1 items=["Snap", "Sequence"] ("Capture mode")
            n132 = event-data() -> ("NewVal"=w491:u16)  [unwired: 1 in, 2 out]
            n133 = call <userlib>:"tm_stopcapture.vi"("error in (no error)"=w498, "Handle in"=w499) -> ("error out"=w496:errorcluster, "Handle out"=w497:u32)  [unwired: 8 in]
            n134 = call <userlib>:"tm_unpreparecapture.vi"("error in (no error)"=w496, "Handle in"=w497) -> ("error out"=w492:errorcluster, "Handle out"=w489:u32)  [unwired: 8 in]
            n135 = call <userlib>:"tm_setparameter_a.vi"("error in (no error)"=w492, "Value in"=w491, "Parameter"=w490, "Handle in"=w489) -> ("error out"=w493:errorcluster, "Handle out"=w494:u32)  [unwired: 6 in]
            n136 = call <userlib>:"tm_getarea_a.vi"("error in (no error)"=w493, "Handle in"=w494) -> ("error out"=w517:errorcluster, "V Offset"=w519:T5, "H Offset"=w518:T5, "Handle out"=w516:u32, "H Width"=w520:T5, "V Width"=w521:T5)  [unwired: 4 in]
            n137 = Unbundle By Name(w518) -> ("Value"=w512:i32, "Minimum"=w515:i32, "Maximum"=w514:i32, "Increment"=w513:i32)
            n138 = Unbundle By Name(w519) -> ("Value"=w502:i32, "Minimum"=w511:i32, "Maximum"=w510:i32, "Increment"=w509:i32)
            n139 = Unbundle By Name(w520) -> ("Value"=w501:i32, "Minimum"=w508:i32, "Maximum"=w507:i32, "Increment"=w506:i32)
            n140 = Unbundle By Name(w521) -> ("Value"=w500:i32, "Minimum"=w505:i32, "Maximum"=w504:i32, "Increment"=w503:i32)
            n141 = property on="H Offset" class="DigNum (strict)"("Value"=w512, "Minimum"=w515, "Maximum"=w514, "Increment"=w513) -> ()  [unwired: 2 in, 2 out]
            n142 = property on="V Offset" class="DigNum (strict)"("Value"=w502, "Minimum"=w511, "Maximum"=w510, "Increment"=w509) -> ()  [unwired: 2 in, 2 out]
            n143 = property on="H Width" class="DigNum (strict)"("Value"=w501, "Minimum"=w508, "Maximum"=w507, "Increment"=w506) -> ()  [unwired: 2 in, 2 out]
            n144 = property on="V Width" class="DigNum (strict)"("Value"=w500, "Minimum"=w505, "Maximum"=w504, "Increment"=w503) -> ()  [unwired: 2 in, 2 out]
            n145 = local write "SHO"(w512) -> ()
            n146 = local write "SVO"(w502) -> ()
            n147 = local write "SHW"(w501) -> ()
            n148 = local write "SVW"(w500) -> ()
            n149 = call <userlib>:"tm_preparecapture.vi"("error in (no error)"=w517, "Capture mode"=w529, "Handle in"=w516) -> ("error out"=w527:errorcluster, "Buffer Info"=w524:T6, "Handle out"=w528:u32)  [unwired: 5 in, 1 out]
            n150 = call <userlib>:"tm_startcapture_b.vi"("error in (no error)"=w527, "Handle in"=w528) -> ("error out"=w526:errorcluster, "Handle out"=w525:u32)  [unwired: 8 in]
          }
          event "H Offset", "H Width", "V Offset", "V Width": Value Change {
            w574 = 1 items=["Snap", "Sequence"] ("Capture mode")
            n151 = event-data() -> ()  [unwired: 1 in, 4 out]
            n152 = call <userlib>:"tm_stopcapture.vi"("error in (no error)"=w536, "Handle in"=w537) -> ("error out"=w534:errorcluster, "Handle out"=w535:u32)  [unwired: 8 in]
            n153 = local read "H Offset"() -> (w540:i32)
            n154 = local read "H Width"() -> (w541:i32)
            n155 = local read "V Offset"() -> (w542:i32)
            n156 = local read "V Width"() -> (w539:i32)
            n157 = call <userlib>:"tm_unpreparecapture.vi"("error in (no error)"=w534, "Handle in"=w535) -> ("error out"=w532:errorcluster, "Handle out"=w533:u32)  [unwired: 8 in]
            n158 = Bundle("H Offset"=w540, "V Offset"=w542, "H Width"=w541, "V Width"=w539) -> (w538:T7)  [unwired: 1 in]
            n159 = call <userlib>:"tm_setarea.vi"("error in (no error)"=w532, "Sub Region"=w538, "Handle in"=w533) -> ("error out"=w543:errorcluster, "Handle out"=w544:u32)  [unwired: 7 in]
            n160 = call <userlib>:"tm_getarea_a.vi"("error in (no error)"=w543, "Handle in"=w544) -> ("error out"=w562:errorcluster, "V Offset"=w564:T5, "H Offset"=w563:T5, "Handle out"=w561:u32, "H Width"=w565:T5, "V Width"=w566:T5)  [unwired: 4 in]
            n161 = Unbundle By Name(w563) -> ("Value"=w557:i32, "Minimum"=w560:i32, "Maximum"=w559:i32, "Increment"=w558:i32)
            n162 = Unbundle By Name(w564) -> ("Value"=w547:i32, "Minimum"=w556:i32, "Maximum"=w555:i32, "Increment"=w554:i32)
            n163 = Unbundle By Name(w565) -> ("Value"=w546:i32, "Minimum"=w553:i32, "Maximum"=w552:i32, "Increment"=w551:i32)
            n164 = Unbundle By Name(w566) -> ("Value"=w545:i32, "Minimum"=w550:i32, "Maximum"=w549:i32, "Increment"=w548:i32)
            n165 = property on="H Offset" class="DigNum (strict)"("Value"=w557, "Minimum"=w560, "Maximum"=w559, "Increment"=w558) -> ()  [unwired: 2 in, 2 out]
            n166 = property on="V Offset" class="DigNum (strict)"("Value"=w547, "Minimum"=w556, "Maximum"=w555, "Increment"=w554) -> ()  [unwired: 2 in, 2 out]
            n167 = property on="H Width" class="DigNum (strict)"("Value"=w546, "Minimum"=w553, "Maximum"=w552, "Increment"=w551) -> ()  [unwired: 2 in, 2 out]
            n168 = property on="V Width" class="DigNum (strict)"("Value"=w545, "Minimum"=w550, "Maximum"=w549, "Increment"=w548) -> ()  [unwired: 2 in, 2 out]
            n169 = local write "SHO"(w557) -> ()
            n170 = local write "SVO"(w547) -> ()
            n171 = local write "SHW"(w546) -> ()
            n172 = local write "SVW"(w545) -> ()
            n173 = call <userlib>:"tm_preparecapture.vi"("error in (no error)"=w562, "Capture mode"=w574, "Handle in"=w561) -> ("error out"=w572:errorcluster, "Buffer Info"=w569:T6, "Handle out"=w573:u32)  [unwired: 5 in, 1 out]
            n174 = call <userlib>:"tm_startcapture_b.vi"("error in (no error)"=w572, "Handle in"=w573) -> ("error out"=w571:errorcluster, "Handle out"=w570:u32)  [unwired: 8 in]
          }
        }
        n175 = Unbundle By Name(w171) -> ("status"=w184:bool)
        n176 = Compound Arithmetic op=OR(w184, "stop", w162) -> (w183:bool)
      }
      n177 = while {
        tunnel: w28 -> [w108]
        shift-right: [w104] -> _
        shift-left: _ -> [w102]
        shift-right: [w100] -> _
        shift-left: _ -> [w101]
        tunnel: w29 -> [w98]
        shift-right: [w96] -> _
        shift-left: _ -> [w95]
        stop <- w103 stop-if-true
        n178 = Dequeue Element(queue=w108, timeout in ms (-1)=1) -> (element=w107:T3)  [unwired: 1 in, 3 out]
        n179 = Unbundle By Name(w107) -> ("Enum"=w106:T1, "Stack Number"=w105:i32)
        "Enum" <- w106
        n180 = Dequeue Element(queue=w98) -> (element=w94:u16[][], timed out?=w97:bool)  [unwired: 2 in, 2 out]
        n181 = case shown="False" w97 {
          tunnel: w94 -> [w110 w112]
          tunnel: [w110 w111] -> w92
          tunnel: [w109 w112] -> w96
          tunnel: w95 -> [w109 w111]
          frame False {
          }
          frame True {
          }
        }
        "Image" <- w92
        n182 = case shown="\"STOP\"" w106 {
          tunnel: w105 -> [_ w130 _ _ _]
          tunnel: [w122 w140 w156 _ _] -> w104
          tunnel: w102 -> [_ w143 w156 _ _]
          tunnel: [FALSE _ _ TRUE _] -> w103
          tunnel: w92 -> [_ w142 _ _ _]
          tunnel: w101 -> [w120 w138 w154 w157 w159]
          tunnel: [w121 w137 w153 w157 w159] -> w100
          tunnel: "Path" -> [w116 _ _ _ _]
          frame "Start Sequence" {
            # "Public tiff library"
            # "Get path and open file"
            n183 = Equal?(x=w116, y=path "") -> (x = y?=w118:bool)
            n184 = case shown="True" w118 {
              tunnel: w116 -> [w123 _]
              tunnel: [w123 w126] -> w115
              frame False {
              }
              frame True {
                n185 = call "File Dialog"("pattern (all files)"=".tiff", "pattern label"="Tiff Image") -> ("selected path"=w126:path)  [unwired: 10 in, 3 out]
              }
            }
            n186 = case shown="False" "AutoIncrement" {
              tunnel: w115 -> [w127 w129]
              tunnel: [w127 w128] -> w114
              frame False {
              }
              frame True {
                n187 = call "4Digit File Incrementer.vi"("path"=w129) -> ("appended path"=w128:path)  [unwired: 10 in]
              }
            }
            n188 = call "libtiff2_open_w.vi"("error in (no error)"=w120, "Input path"=w114) -> ("error out"=w121:errorcluster, "handle"=w122:i32)  [unwired: 8 in]
            n189 = local write "Path"(w114) -> ()
          }
          frame "Collecting" {
            w146 = T8 7 items=["Grayscale (U8)", "Grayscale (I16)", "Grayscale (SGL)", "Complex (CSG)", "RGB (U32)", "HSL (U32)", "RGB (U64)", "Grayscale (U16)"] ("Image Type")
            # "Add Image to write scan line"
            n190 = Number To Decimal String(number=w130) -> (decimal integer string=w131:string)  [unwired: 1 in]
            n191 = call "IMAQ Create"("Image Name"="Sim Stack", "Image Type"=w146) -> ("New Image"=w135:T9)  [unwired: 3 in, 1 out]
            n192 = call "IMAQ Write Custom Data"("Custom Data In"=w131, "Key"="test", "Image"=w135) -> ("error out"=w133:errorcluster, "Image Out"=w134:T9)  [unwired: 7 in]
            n193 = call "IMAQ ArrayToImage"("Image Pixels (U16)"=w142, "error in (no error)"=w133, "Image"=w134) -> ("Image Out"=w144:T9)  [unwired: 7 in, 1 out]
            n194 = call "libtiff2_writeScanLine_U16.vi"("error in (no error)"=w138, "page"=w130, "Image"=w144, "Handle"=w143) -> ("error out"=w141:errorcluster, "Handle out"=w140:i32)  [unwired: 6 in]
            n195 = case shown="Error" w141 {
              selector: w141 -> [w147 w149]
              tunnel: w140 -> [_ w150]
              tunnel: [w147 w148] -> w137
              frame No Error {
              }
              frame Error {
                n196 = call "libtiff2_close.vi"("error in (no error)"=w149, "Handle"=w150) -> ("error out"=w148:errorcluster)  [unwired: 8 in]
              }
            }
            n197 = property on="Capture" class="Bool (strict)"("DisabledEnum"=T2."Disabled and Grayed Out" ("Disabled"), "BoolText.Text"="Saving" ("Boolean Text.Text")) -> ()  [unwired: 2 in, 2 out]
          }
          frame "End" {
            (unwired) FALSE
            # "Close image file, reset capturing button"
            n198 = call "libtiff2_close.vi"("error in (no error)"=w154, "Handle"=w156) -> ("error out"=w155:errorcluster)  [unwired: 8 in]
            n199 = property on="Capture" class="Bool (strict)"(error in=w155, "BoolText.Text"="OK" ("Boolean Text.Text"), "DisabledEnum"=T2."Enabled" ("Disabled")) -> (error out=w153:errorcluster)  [unwired: 1 in, 1 out]
          }
          frame "STOP" {
          }
          frame "Idle" {
          }
        }
      }
      n200 = call <userlib>:"tm_stopcapture.vi"("error in (no error)"=w59, "Handle in"=w60) -> ("error out"=w56:errorcluster, "Handle out"=w57:u32)  [unwired: 8 in]
      n201 = call <userlib>:"tm_unpreparecapture.vi"("error in (no error)"=w56, "Handle in"=w57) -> ("error out"=w55:errorcluster, "Handle out"=w58:u32)  [unwired: 8 in]
      n202 = call <userlib>:"tm_closecamera.vi"("error in (no error)"=w55, "Handle in"=w58) -> ("error out"=w89:errorcluster)  [unwired: 9 in]
      n203 = call <userlib>:"tm_deinitialize.vi"("error in (no error)"=w89) -> ("error out"=w88:errorcluster)  [unwired: 10 in]
    }
  }
  "error out" <- w3
